vi "PXI_Host_FXP_Read_NewMethod_Benchmark.vi"() -> ()   [LabVIEW 2018]
uses:
  cRIO RT/FPGA Bitfile Register Operations/Scalar IO Operations/TypeDefs/FXP Configuration.ctl
  <vilib>/fxp/LVFixedPointRepBitsTypeDef.ctl
  <vilib>/fxp/LVFixedPointRepRangeTypeDef.ctl
  <vilib>/FPGAPlugInAG/Dynamic/niLvFpga_Close_Dynamic.vi
  <vilib>/rvi/interface/nirviCloseFPGA/nirviCloseFPGA.xnode
  cRIO RT/FPGA Bitfile Register Operations/Scalar IO Operations/Read Methods/Read Data Register/Instances/Read FXP.vi
  cRIO RT/FPGA Bitfile Register Operations/Scalar IO Operations/FPGA Register IO.lvlib
panel:
  out "DBL Value":dbl
  out "error out":errorcluster
  out "Execution time (s)":dbl
  # "Recorded time"
  # "3.37551E-5"
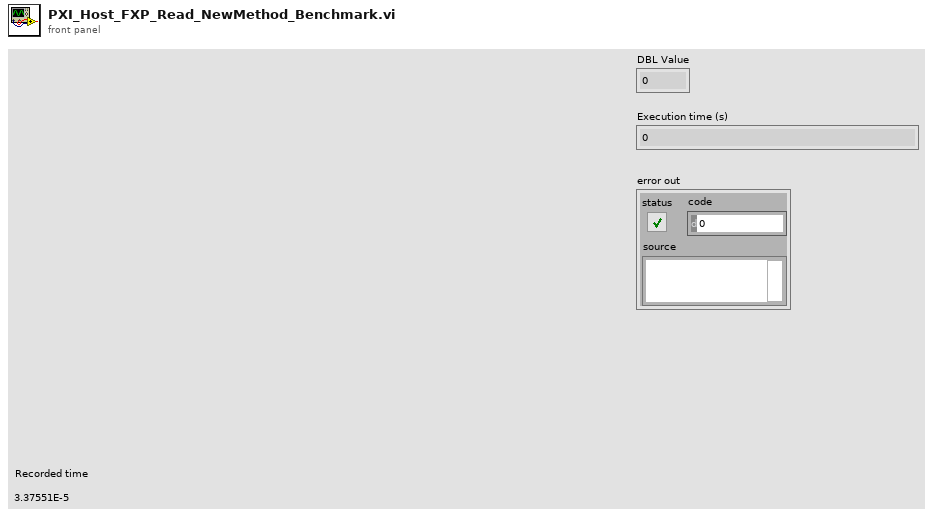
[diagram p1: front panel]
types:
  T1 = typedef "FPGA Register IO.lvlib/FXP Configuration.ctl" = cluster{"FXP Representation":T2, "FXP Range":T3}
  T2 = typedef "LVFixedPointRepBitsTypeDef.ctl" = cluster{"Signed":bool, "Word Length":u32, "Integer Word Length":i32}
  T3 = typedef "LVFixedPointRepRangeTypeDef.ctl" = cluster{"Range Min":dbl, "Range Max":dbl, "Delta":dbl}
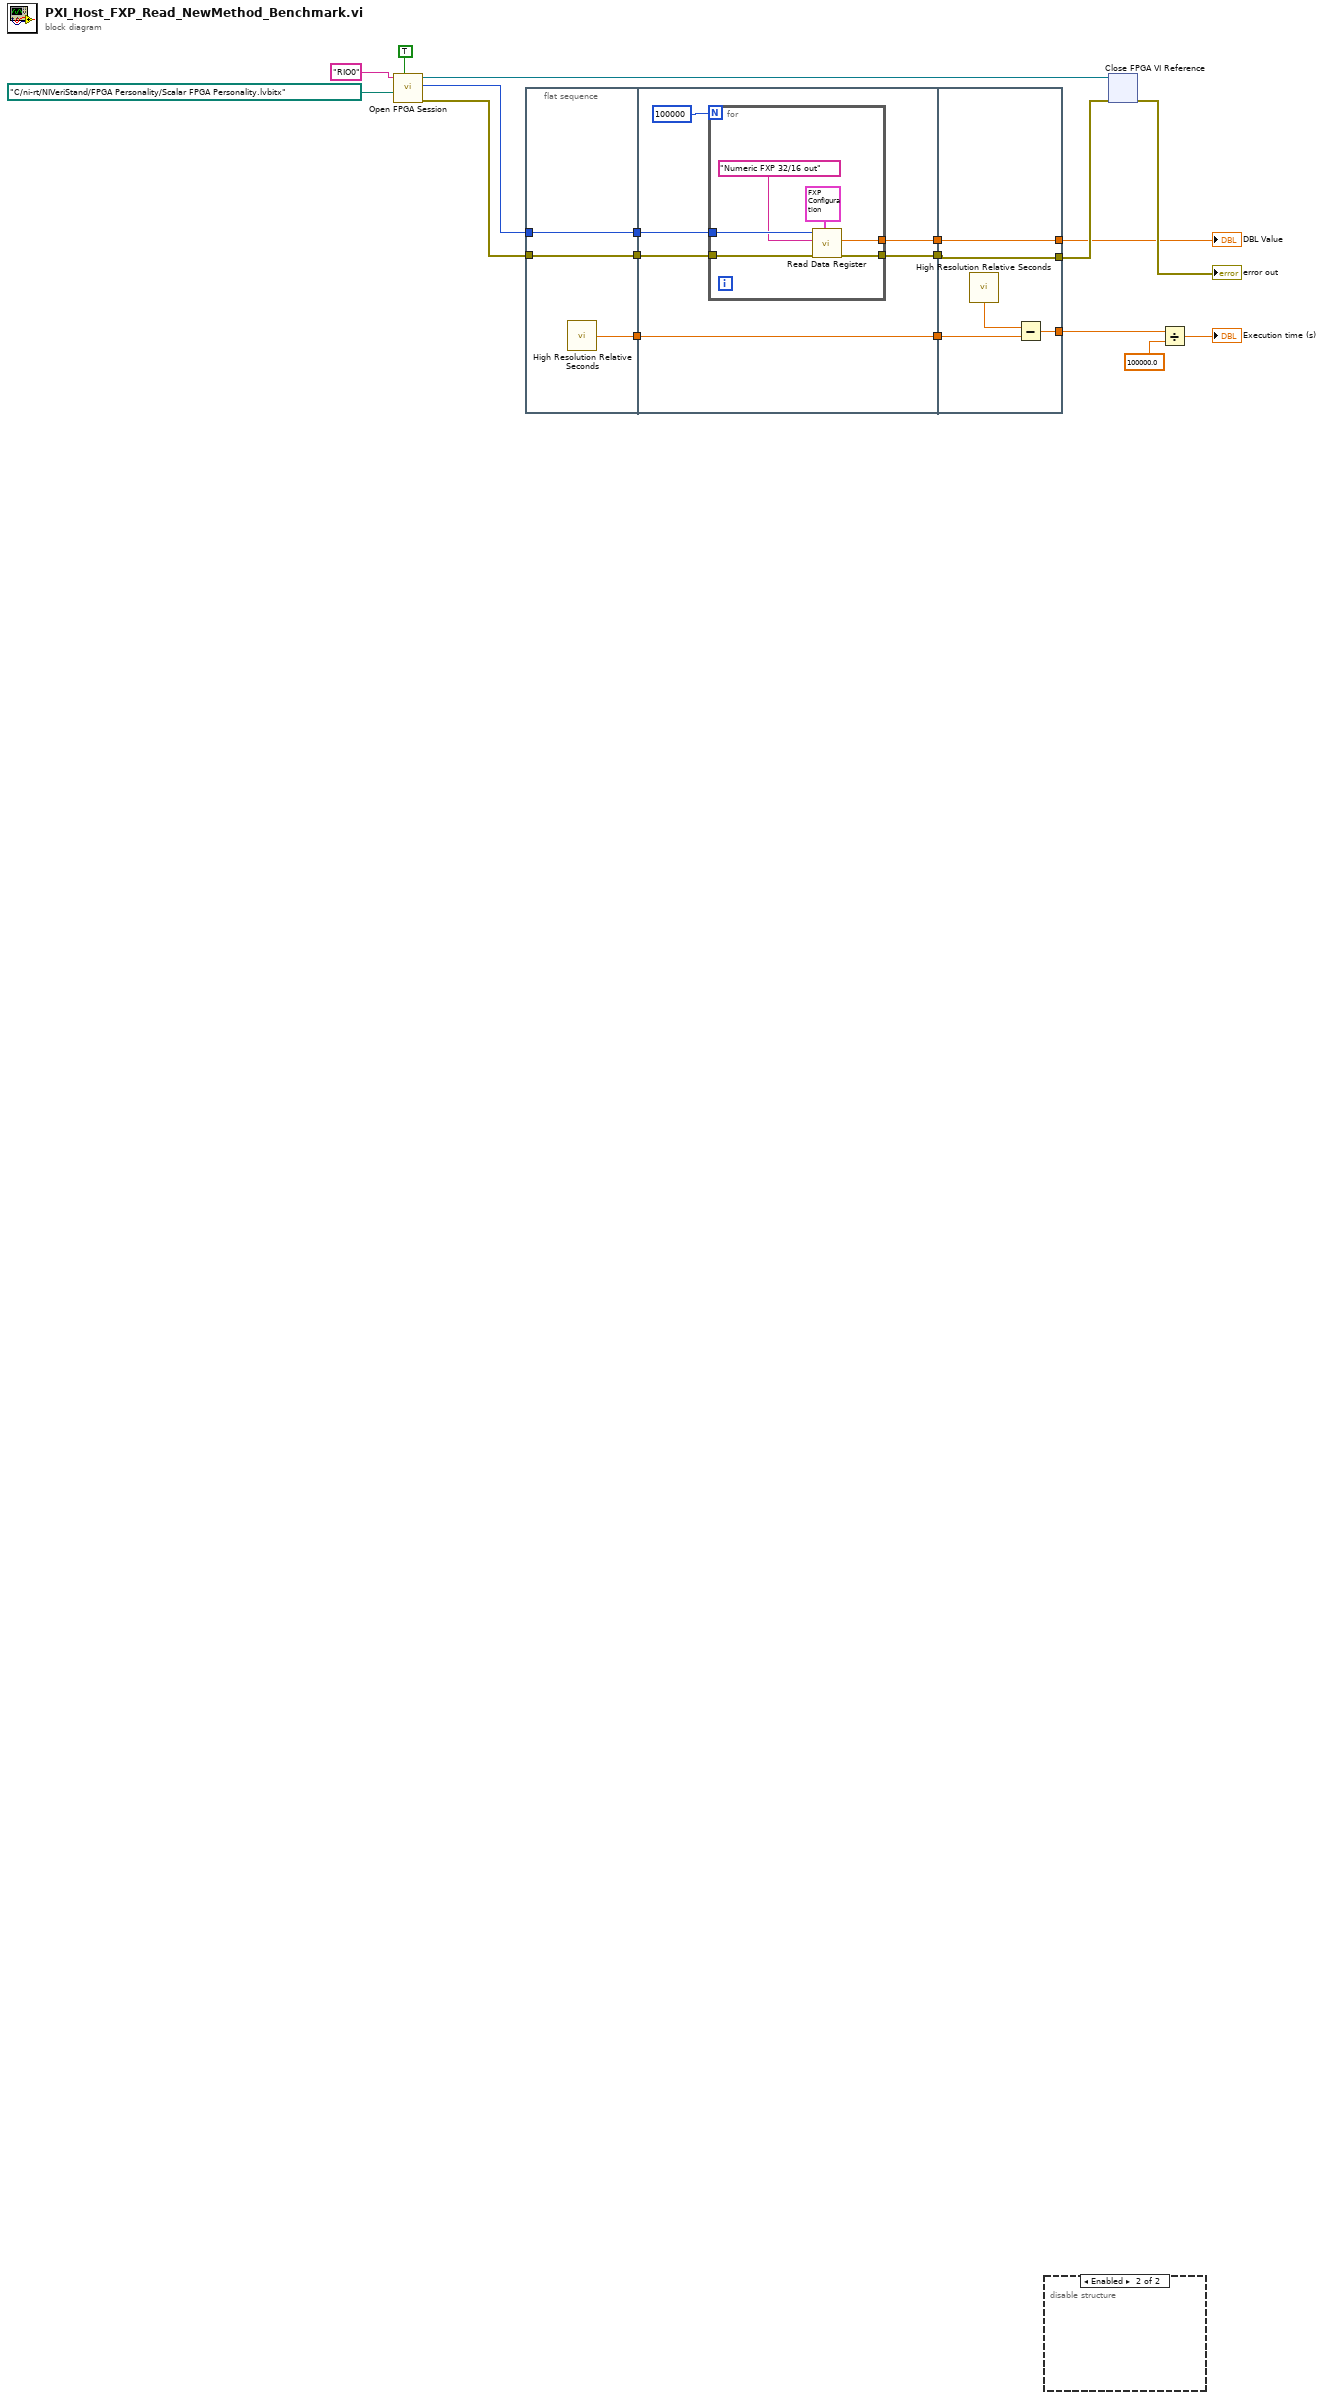
[diagram p0: block diagram]
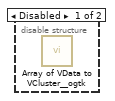
[diagram p2: hidden frame]
diagram:
  n1 = call "Open FPGA Session.vi"("run when loaded (T)"=TRUE, "bitfile path"=path "C:/ni-rt/NIVeriStand/FPGA Personality/Scalar FPGA Personality.lvbitx", "device address"="RIO0") -> ("error out"=w12:errorcluster, "session out"=w16:u32, "bitfile reference out"=w11:refnum<k20>)  [unwired: 6 in]
  n2 = flat-sequence {
    tunnel: [w21] -> w5
    tunnel: w16 -> [w20]
    tunnel: [w20] -> w4
    tunnel: w12 -> [w19]
    tunnel: [w19] -> w6
    tunnel: [w26] -> w3
    tunnel: w5 -> [w26]
    tunnel: w4 -> [w25]
    tunnel: w6 -> [w24]
    tunnel: [w23] -> w2
    tunnel: [w22] -> w1
    tunnel: w3 -> [w37]
    tunnel: [w36] -> w18
    tunnel: w2 -> [w35]
    tunnel: [w35] -> w10
    tunnel: w1 -> [w34]
    tunnel: [w34] -> w8
    frame #0 {
      n3 = call <vilib>:"High Resolution Relative Seconds.vi"() -> ("relative seconds"=w21:dbl)
    }
    frame #1 {
      n4 = for {
        N: 100000 -> [_]
        tunnel: w25 -> [w33]
        tunnel: w24 -> [w31]
        tunnel: [w30] -> w23
        tunnel: [w29] -> w22
        n5 = call-poly "Read Data Register.vi"("FXP Configuration"=T1 {"FXP Representation"={"Signed"=TRUE, "Word Length"=32, "Integer Word Length"=16}, "FXP Range"={"Range Min"=-32768.0, "Range Max"=32767.999985, "Delta"=1.52588e-05}}, "error in"=w31, "register name"="Numeric FXP 32/16 out", "session in"=w33) -> ("error out"=w30:errorcluster, "DBL Value"=w29:dbl)  [unwired: 5 in, 1 out]
      }
    }
    frame #2 {
      n6 = call <vilib>:"High Resolution Relative Seconds.vi"() -> ("relative seconds"=w38:dbl)
      n7 = Subtract(x=w38, y=w37) -> (x-y=w36:dbl)
    }
  }
  n8 = disable-structure shown="Enabled" {
    frame Disabled {
      n9 = call <userlib>:"Array of VData to VCluster__ogtk.vi"() -> ()  [unwired: 10 in, 2 out]
    }
    frame Enabled {
    }
  }
  n10 = xnode "Close FPGA VI Reference"("FPGA VI Reference In"=w11, "error in"=w10) -> ("error out"=→"error out":errorcluster)
  n11 = Divide(x=w18, y=100000.0) -> (x/y=→"Execution time (s)":dbl)
  "DBL Value" <- w8
